vi "Outputs.vi"(8 "error in (no error)":errorcluster, 11 "State in":T1={"State"=enum."Idle", "Start Time"=timestamp(0 s since 1904-01-01), "Configuration"={"Cycle Period"=0.0, "Manual Entry"=0.0, "Output Device"=enum."Default", "EPOS4 Settings"={"VISA resource name"="", "axis"={"keyHandle"=1, "nodeId"=1}, "Simulated?"=FALSE}}, "Current Time"=timestamp(0 s since 1904-01-01), "First Iteration"=FALSE, "Data"={"Centrifuge Speed"=0.0}, "Process Name"="", "Centrifuge On?"=enum."Off", "Output Error"=FALSE, "Log Started"=FALSE}) -> (0 "error out":errorcluster, 3 "State out":T1={"State"=enum."Idle", "Start Time"=timestamp(0 s since 1904-01-01), "Configuration"={"Cycle Period"=0.0, "Manual Entry"=0.0, "Output Device"=enum."Default", "EPOS4 Settings"={"VISA resource name"="", "axis"={"keyHandle"=1, "nodeId"=1}, "Simulated?"=FALSE}}, "Current Time"=timestamp(0 s since 1904-01-01), "First Iteration"=FALSE, "Data"={"Centrifuge Speed"=0.0}, "Process Name"="", "Centrifuge On?"=enum."Off", "Output Error"=FALSE, "Log Started"=FALSE})   [LabVIEW 2018, in "Centrifuge Module.lvlib" / "Centrifuge Module Engine.lvlib"]
uses:
  Centrifuge Module Engine.lvlib
  State Cluster.ctl
  State Enum.ctl
  Centrifuge Module Settings Cluster.ctl
  EPOS4/Controls/Device Selection.ctl
  EPOS4/Controls/EPOS Communication Settings.ctl
  Tag VIs/Tag FGV Operation Enum.ctl
  Shared Variables/Dynamic Shared Variables.lvlib
  EPOS4/EPOS4.lvlib
  Centrifuge Module.lvlib
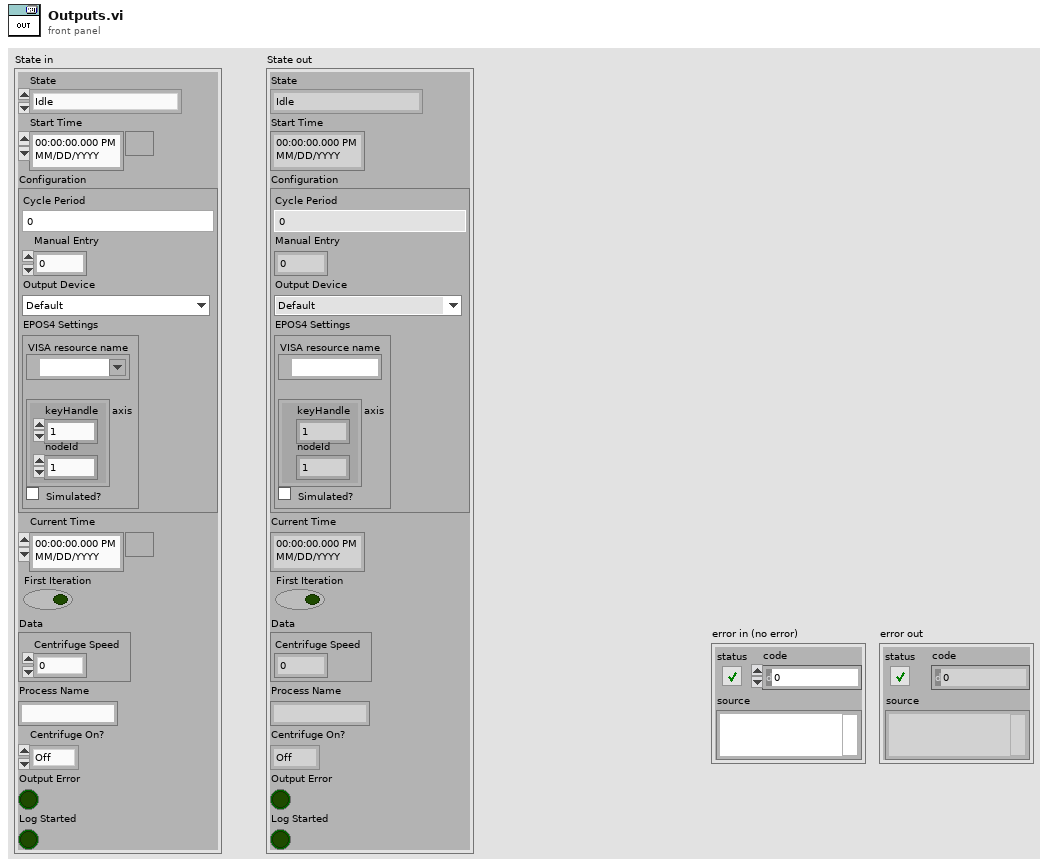
[diagram p1: front panel]
types:
  T1 = typedef "Centrifuge Module.lvlib/Centrifuge Module Engine.lvlib/State Cluster.ctl" = cluster{"State":T2, "Start Time":timestamp, "Configuration":T3, "Current Time":timestamp, "First Iteration":bool, "Data":cluster{"Centrifuge Speed":dbl}, "Process Name":string, "Centrifuge On?":enum16{"Off", "On", "Not Initialized"}, "Output Error":bool, "Log Started":bool}
  T2 = typedef "Centrifuge Module.lvlib/Centrifuge Module Engine.lvlib/State Enum.ctl" = enum16{"Measuring", "Idle", "Paused"}
  T3 = typedef "Centrifuge Module.lvlib/Centrifuge Module Settings Cluster.ctl" = cluster{"Cycle Period":dbl, "Manual Entry":dbl, "Output Device":T4, "EPOS4 Settings":T5}
  T4 = typedef "Device Selection.ctl" = enum16{"Default", "EPOS4"}
  T5 = typedef "EPOS4.lvlib/EPOS Communication Settings.ctl" = cluster{"VISA resource name":refnum<visa-resource-name>, "axis":cluster{"keyHandle":u32, "nodeId":u16}, "Simulated?":bool}
  T6 = typedef "Tag FGV Operation Enum.ctl" = enum16{"Init", "Set Notification Queue", "Create Tag", "Commit", "Write Tag (Numeric)", "Write Tag (Boolean)", "Read All Tags", "Read One Tag", "Delete Tag Category", "Set Alarm Parameters (Numeric)", "Set Alarm Parameters (Boolean)", "Enable All Alarms", "Disable All Alarms", "Delete All Tags", "Read Alarms", "Ack Alarm", "Read Alarm Parameters (Numeric)", "Read Alarm Parameters (Boolean)"}
  T7 = typedef "Centrifuge Module.lvlib/Centrifuge Module Tag Names Cluster.ctl" = cluster{"Centrifuge Speed":string, "Output Device Tag":string}
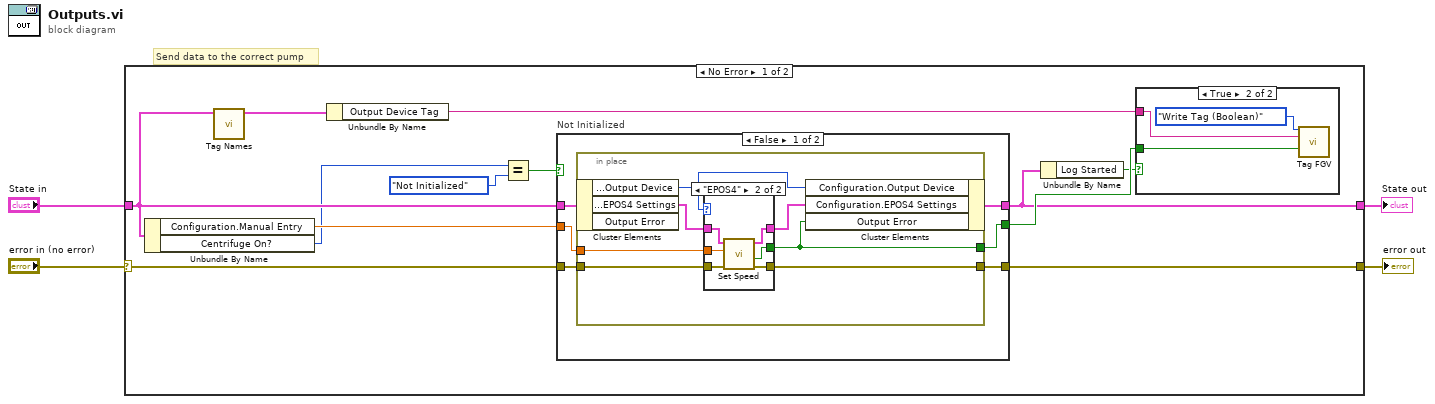
[diagram p0: block diagram]
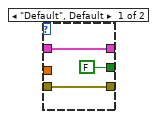
[diagram p3: hidden frame]
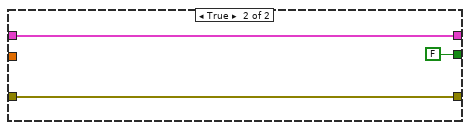
[diagram p4: hidden frame]
diagram:
  # "Send data to the correct pump"
  n1 = case shown="No Error" "error in (no error)" {
    selector: "error in (no error)" -> [w16 w46]
    tunnel: [w14 w46] -> w3
    tunnel: "State in" -> [w8 w45]
    tunnel: [w7 w45] -> w1
    frame No Error {
      n2 = Unbundle By Name(w8) -> ("Configuration.Manual Entry"=w9:dbl, "Centrifuge On?"=w5:enum16{"Off", "On", "Not Initialized"})
      n3 = call "Tag Names.vi"("State In"=w8) -> ("Centrifuge Module Tag Names"=w15:T7)  [unwired: 8 in, 2 out]
      n4 = Unbundle By Name(w15) -> ("Output Device Tag"=w13:string)
      n5 = Equal?(x=w5, y=enum16{"Off", "On", "Not Initialized"}."Not Initialized" ("x")) -> (x = y?=w11:bool)
      n6 = case "Not Initialized" shown="False" w11 {
        tunnel: w16 -> [w25 w43]
        tunnel: [w24 w43] -> w14
        tunnel: [w22 FALSE ("Connection Error")] -> w12
        tunnel: w9 -> [w23 _]
        tunnel: w8 -> [w21 w42]
        tunnel: [w20 w42] -> w7
        frame False {
          n7 = in-place {
            in-place-border: w25 -> [w32]
            in-place-border: [w31] -> w24
            in-place-border: w23 -> [w30]
            in-place-border: [w27] -> w22
            n8 = in-place-cluster #1(w21) -> ("Configuration.Output Device"=w26:T4, "Configuration.EPOS4 Settings"=w29:T5)  [unwired: 1 out]
            n9 = case shown="\"EPOS4\"" w26 {
              tunnel: w32 -> [w35 w39]
              tunnel: [w35 w38] -> w31
              tunnel: w30 -> [_ w40]
              tunnel: w29 -> [w34 w41]
              tunnel: [FALSE ("Connection Error") w37] -> w27
              tunnel: [w34 w36] -> w28
              frame "Default", Default {
              }
              frame "EPOS4" {
                n10 = call "Set Speed.vi"("error in (no error)"=w39, "speed"=w40, "EPOS4 Settings In"=w41) -> ("error out"=w38:errorcluster, "Connection Error"=w37:bool, "EPOS4 Settings Out"=w36:T5)  [unwired: 6 in]
              }
            }
            n11 = in-place-cluster #1("Configuration.Output Device"=w26, "Configuration.EPOS4 Settings"=w28, "Output Error"=w27) -> (w20:T1)
          }
        }
        frame True {
        }
      }
      n12 = Unbundle By Name(w7) -> ("Log Started"=w10:bool)
      n13 = case shown="True" w10 {
        tunnel: w13 -> [_ w19]
        tunnel: w12 -> [_ w18]
        frame False {
        }
        frame True {
          n14 = call "Tag FGV.vi"("Operation"=Tag_FGV_Operation_Enum."Write Tag (Boolean)", "Tag Name"=w19, "Data"=w18) -> ()  [unwired: 5 in, 8 out]
        }
      }
    }
    frame Error {
    }
  }
  "error out" <- w3
  "State out" <- w1
